vi "test_regex filter.vi"(7 "regexes":string[](array[string]), 8 "error in":errorcluster, 9 "aggregation method":T1, 10 "match behavior":T2, 11 "directory":path=path "C:/Users/Colin/Documents/software_projects/labview/glog/logs/test") -> (0 "error out":errorcluster, 3 "failure info":T3 {"Log Record"."timestamp" format="%<%x %.3X>T"})   [LabVIEW 2018]
uses:
  src/api/logger_class/Failure Information.ctl
  src/api/logger_class/Log Record.ctl
  src/api/logger_class/Internal Log Levels.ctl
  src/api/extension/filter_interface/Match Behavior.ctl
  src/api/extension/filter_interface/Aggregation Method.ctl
  src/api/logger_class/Log Levels.ctl
  src/api/configuration/filters/regex_filter/Regex.lvclass
  C:/Users/Colin/Documents/software_projects/labview/glog/src/api/extension/filter_interface/Filter.lvclass
  src/api/configuration/handlers/file_handler/File Handler.lvclass
  C:/Users/Colin/Documents/software_projects/labview/glog/src/api/extension/formatting_handler_interface/Formatting Handler.lvclass
  src/api/configuration/filters/regex_filter/New (Array).vi
  src/api/logger_class/Log (Parts).vi
  src/api/logger_class/Logger.lvclass
  src/api/GLog.lvlib
panel:
  # "Connector Pane"
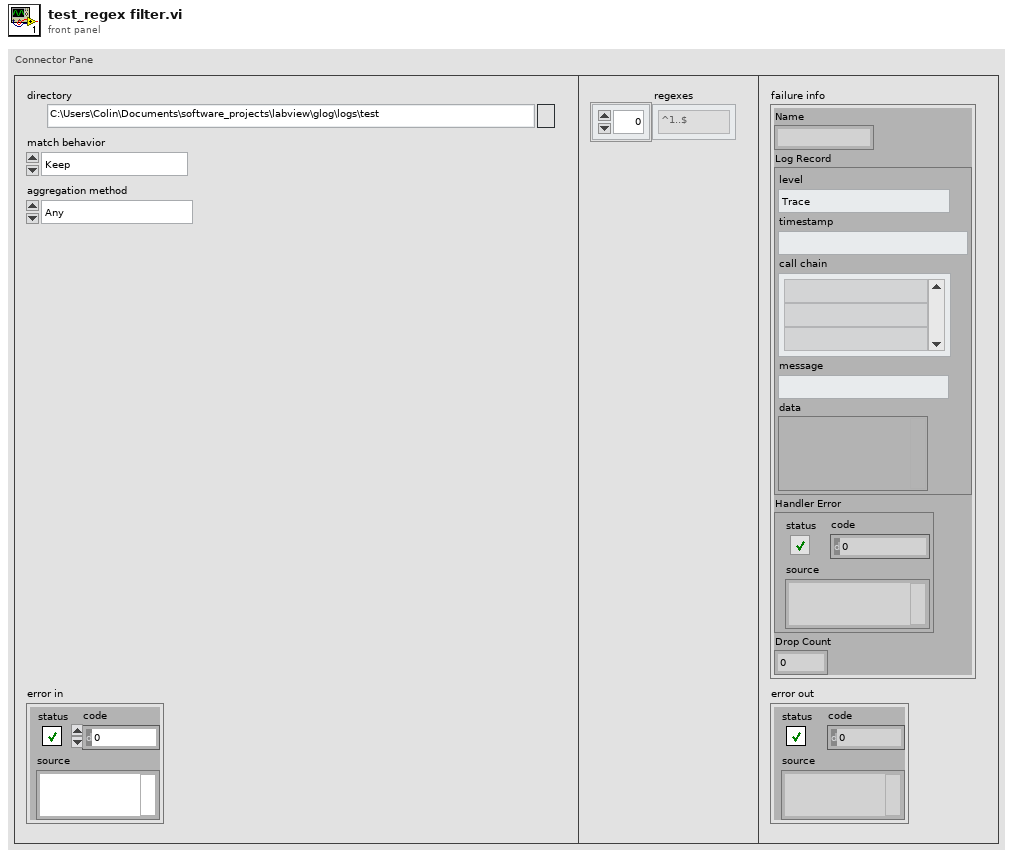
[diagram p1: front panel]
types:
  T1 = typedef "GLog.lvlib/Aggregation Method.ctl" = enum16{"Any", "Only", "All", "None"}
  T2 = typedef "GLog.lvlib/Match Behavior.ctl" = enum16{"Keep", "Discard"}
  T3 = typedef "GLog.lvlib/Logger.lvclass/Failure Information.ctl" = cluster{"Name":string, "Log Record":T4, "Handler Error":errorcluster, "Drop Count":u32}
  T4 = typedef "GLog.lvlib/Logger.lvclass/Log Record.ctl" = cluster{"level":T5, "timestamp":timestamp, "call chain":string[], "message":string, "data":variant}
  T5 = typedef "GLog.lvlib/Logger.lvclass/Internal Log Levels.ctl" = enum16{"Trace", "Debug", "Info", "Warning", "Error", "Critical", "Internal"}
  T6 = typedef "GLog.lvlib/Logger.lvclass/Log Levels.ctl" = enum16{"Trace", "Debug", "Info", "Warning", "Error", "Critical"}
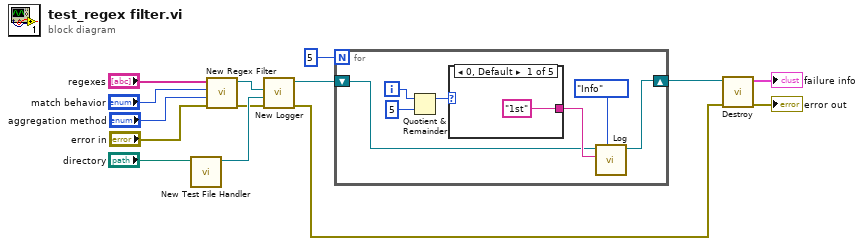
[diagram p0: block diagram]
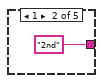
[diagram p2: hidden frame]
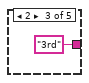
[diagram p3: hidden frame]
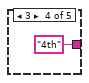
[diagram p4: hidden frame]
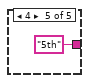
[diagram p5: hidden frame]
diagram:
  n1 = call "New Test File Handler.vi"("log directory"="directory") -> ("test file handler"=w12:refnum<class "File Handler.lvclass">)  [unwired: 10 in]
  n2 = call-poly "New Regex Filter.vi"("error in (no error)"="error in", "aggregation method (all)"="aggregation method", "match behavior (keep)"="match behavior", "regex strings"="regexes") -> ("error out"=w8:errorcluster, "regex out"=w1:refnum<class "Regex.lvclass">)  [unwired: 6 in]
  n3 = call "New Logger.vi"("error in (no error)"=w8, "log handler (file handler)"=w12, "log filter (none)"=w1) -> ("error out"=w11:errorcluster, "logger"=w2:refnum<class "Logger.lvclass">)  [unwired: 7 in]
  n4 = for {
    N: 5 -> [_]
    shift-right: [w17] -> w3
    shift-left: w2 -> [w16]
    i -> [w18]
    n5 = Quotient & Remainder(x=w18, y=5) -> (x-y*floor(x/y)=w20:i32)  [unwired: 1 out]
    n6 = case shown="0, Default" w20 {
      tunnel: ["1st" ("message") "2nd" ("message") "3rd" ("message") "4th" ("message") "5th" ("message")] -> w19
      frame 0, Default {
      }
      frame 1 {
      }
      frame 2 {
      }
      frame 3 {
      }
      frame 4 {
      }
    }
    n7 = call-poly "Log.vi"("log level"=Log_Levels."Info", "message"=w19, "logger in"=w16) -> ("logger out"=w17:refnum<class "Logger.lvclass">)  [unwired: 8 in]
  }
  n8 = call "Destroy.vi"("error in (no error)"=w11, "logger in"=w3) -> ("error out"=→"error out":errorcluster, "failure info"=→"failure info":T3)  [unwired: 8 in]
